vi "CPP-6068SpectralAnalysis.vi"() -> (5 "Plug in titles":string[](array[string]), 7 "Plug in values":string[](array[string]))   [LabVIEW 2011]
uses:
  Globals/Meas_global.vi
panel:
  out "BlockStartTime":dbl format="%#_12f"
  out "Titles":string[](array[string])
  out "Results":dbl[][](array[numeric]) format="%#_3g"
  in  "SearchBands":cluster{"Min":dbl, "Max":dbl, "Name":string}[](array[cluster])=[{"Min"=40.0, "Max"=70.0, "Name"=""}, {"Min"=100.0, "Max"=140.0, "Name"=""}, {"Min"=450.0, "Max"=510.0, "Name"=""}, {"Min"=600.0, "Max"=680.0, "Name"=""}]
  out "TimeRunStarted":dbl format="%<%H:%M:%S\n%x %Z>T"
  out "Processing last block?":bool
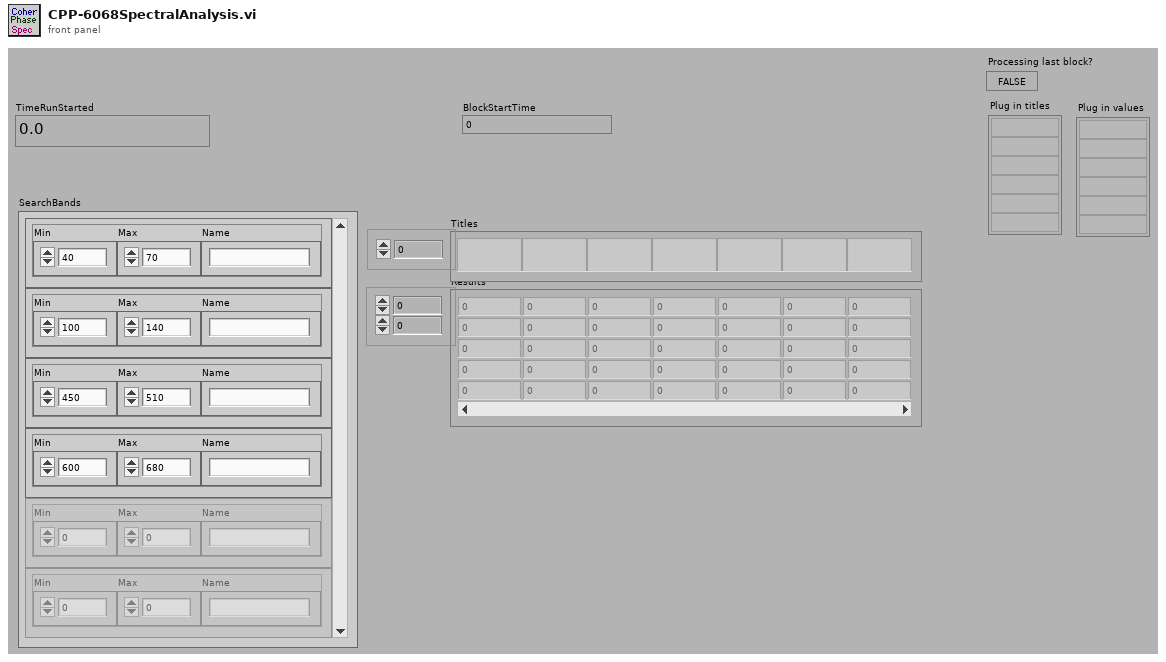
[diagram p1: front panel]
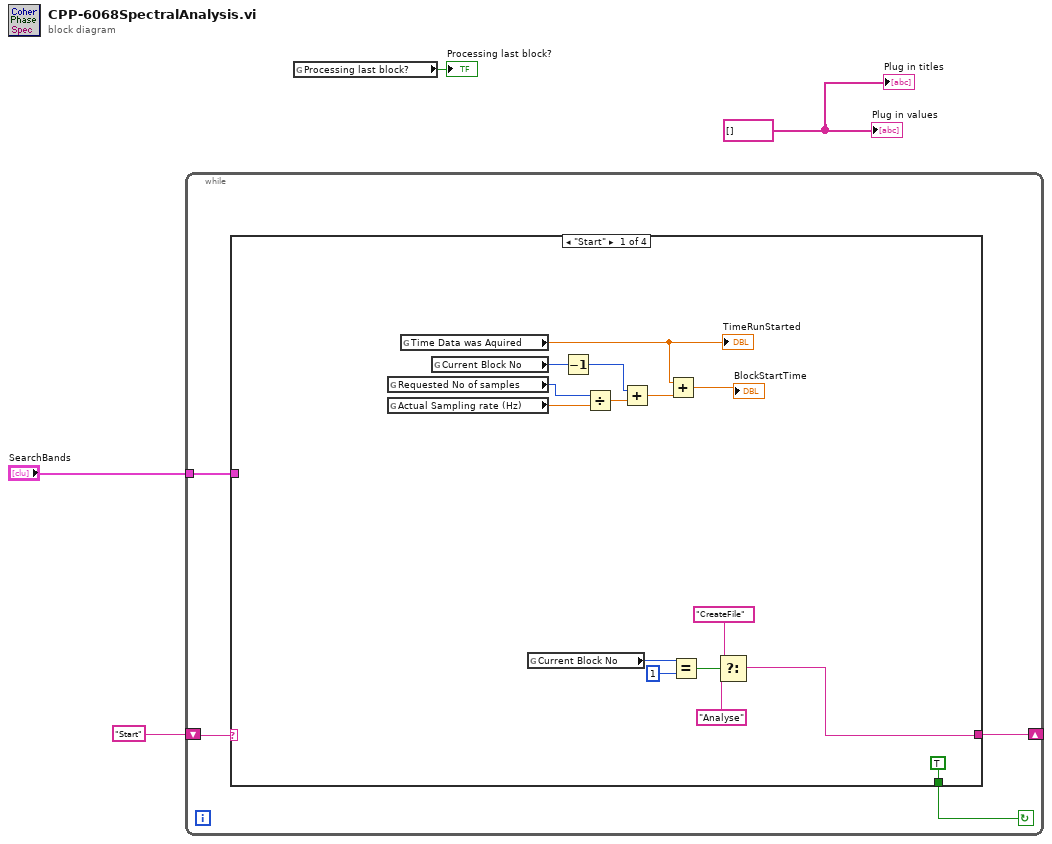
[diagram p0: block diagram]
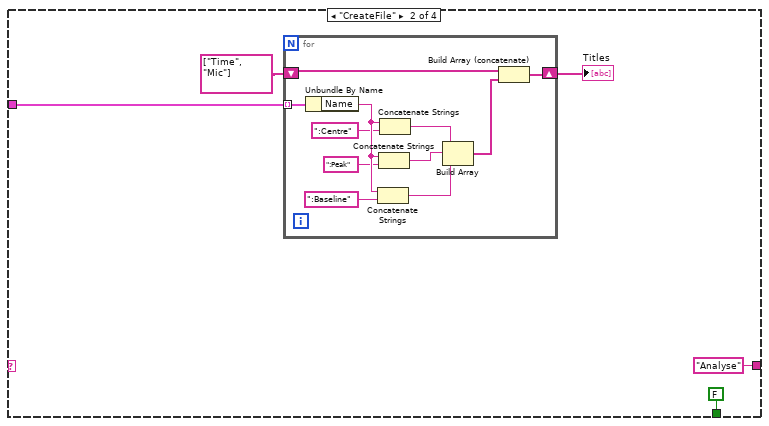
[diagram p2: hidden frame]
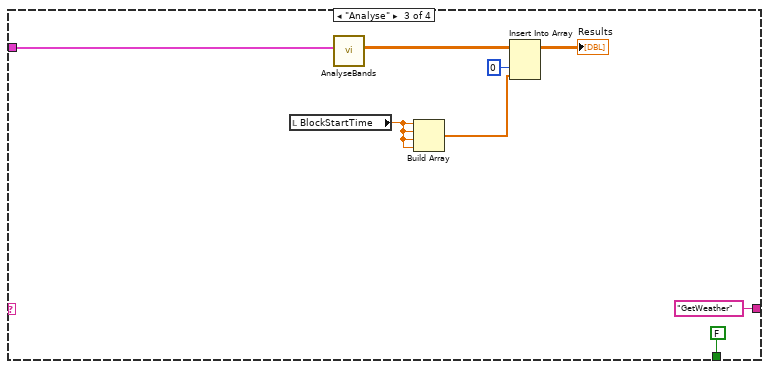
[diagram p3: hidden frame]
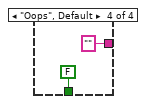
[diagram p4: hidden frame]
diagram:
  w3 = string[] [] ("Add in values")
  n1 = while {
    tunnel: "SearchBands" -> [w8]
    shift-right: [w6] -> _
    shift-left: "Start" -> [w7]
    stop <- w5 continue-if-true
    n2 = case shown="\"Start\"" w7 {
      tunnel: w8 -> [_ w26 w43 _]
      tunnel: [w20 "Analyse" "GetWeather" ""] -> w6
      tunnel: [TRUE FALSE FALSE FALSE] -> w5
      frame "Start" {
        n3 = global read "Meas_global.vi" "Requested No of samples"() -> (w15:i32)
        n4 = global read "Meas_global.vi" "Actual Sampling rate (Hz)"() -> (w14:dbl)
        n5 = global read "Meas_global.vi" "Time Data was Aquired"() -> (w10:dbl)
        "TimeRunStarted" <- w10
        n6 = global read "Meas_global.vi" "Current Block No"() -> (w16:i32)
        n7 = global read "Meas_global.vi" "Current Block No"() -> (w23:i32)
        n8 = Decrement(x=w16) -> (x-1=w12:i32)
        n9 = Divide(x=w15, y=w14) -> (x/y=w13:dbl)
        n10 = Add(x=w12, y=w13) -> (x+y=w11:dbl)
        n11 = Add(x=w10, y=w11) -> (x+y=→"BlockStartTime":dbl)
        n12 = Equal?(x=w23, y=1) -> (x = y?=w21:bool)
        n13 = Select(t="CreateFile", s=w21, f="Analyse") -> (s? t:f=w20:string)
      }
      frame "CreateFile" {
        n14 = for {
          shift-right: [w29] -> w28
          shift-left: string[] ["Time", "Mic"] -> [w30]
          tunnel: w26 -> [w39] mode=indexing
          n15 = Unbundle By Name(w39) -> ("Name"=w38:string)
          n16 = Concatenate Strings(w38, ":Baseline" ("string")) -> (w32:string)
          n17 = Concatenate Strings(w38, ":Peak" ("string")) -> (w33:string)
          n18 = Concatenate Strings(w38, ":Centre" ("string")) -> (w34:string)
          n19 = Build Array(w34, w33, w32) -> (w31:string[])
          n20 = Build Array (concatenate)(w30, w31) -> (w29:string[])
        }
        "Titles" <- w28
      }
      frame "Analyse" {
        n21 = local read "BlockStartTime"() -> (w40:dbl)
        n22 = call "AnalyseBands.vi"("SearchBands"=w43) -> ("Results"=w47:dbl[][])  [unwired: 10 in]
        n23 = Build Array(w40, w40, w40, w40) -> (w45:dbl[])
        n24 = Insert Into Array(array=w47, index (col)=0 ("disabled index (col)"), new element=w45) -> (→"Results":dbl[][])  [unwired: 1 in]
      }
      frame "Oops", Default {
      }
    }
  }
  n25 = global read "Meas_global.vi" "Processing last block?"() -> (→"Processing last block?":bool)
  "Plug in titles" <- w3
  "Plug in values" <- w3
